vi "Spec - Set LabVIEW Compatibility String.vi"(8 "error in (no error)":errorcluster, 10 "Exclusive_LabVIEW_Version":string, 11 "spec path":path) -> (0 "error out":errorcluster)   [LabVIEW 2015]
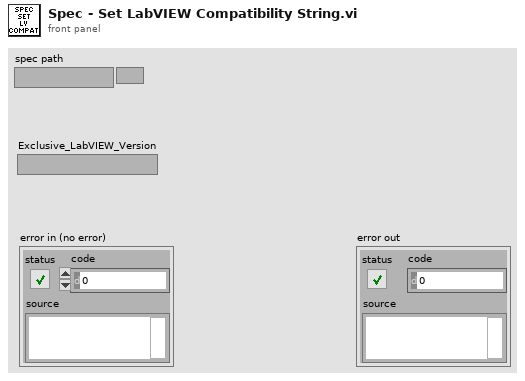
[diagram p1: front panel]
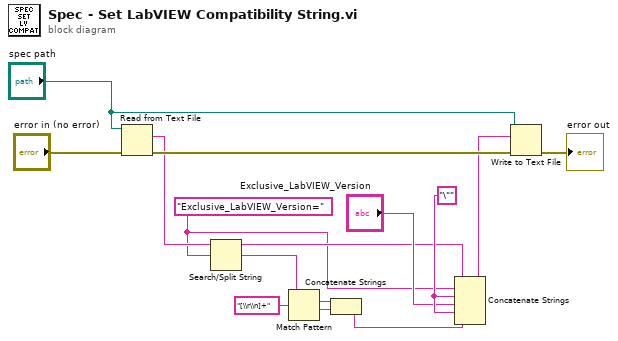
[diagram p0: block diagram]
diagram:
  w4 = "\"" ("search string/char (-)")
  w1 = "Exclusive_LabVIEW_Version=" ("search string/char (-)")
  n1 = Read from Text File(file (use dialog)="spec path", error in="error in (no error)") -> (text=w10:string, error out=w14:errorcluster)  [unwired: 2 in, 2 out]
  n2 = Search/Split String(string=w10, search string/char (-)=w1) -> (substring before match=w2:string, match + rest of string=w5:string)  [unwired: 1 in, 1 out]
  n3 = Match Pattern(string=w5, regular expression="[\\r\\n]+") -> (match substring=w7:string, after substring=w8:string)  [unwired: 1 in, 2 out]
  n4 = Concatenate Strings(w7, w8) -> (w9:string)
  n5 = Concatenate Strings(w2, w1, w4, "Exclusive_LabVIEW_Version", w4, w9) -> (w11:string)
  n6 = Write to Text File(file (use dialog)="spec path", text=w11, error in=w14) -> (error out=→"error out":errorcluster)  [unwired: 1 in, 2 out]
